vi "ATSh_SetTriggerDelay.vi"(10 "Delay":u32, 11 "Handle":u32) -> (0 "Return Code":u32, 3 "Handle_Out":u32)   [LabVIEW 2010]
doc: "_____AlazarTech, Scope_____\n\nConfigure the Trigger delay circuitry.\nHandle input."
uses:
  ATSApi.dll
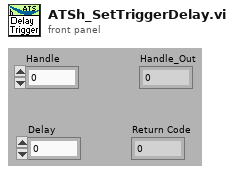
[diagram p1: front panel]
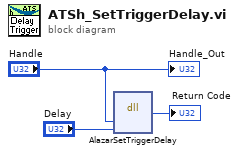
[diagram p0: block diagram]
diagram:
  n1 = dll-call lib="ATSApi.dll" fn="AlazarSetTriggerDelay"("h"="Handle", "Delay"="Delay") -> (→"Return Code":u32)  [unwired: 5 in, 2 out]
  "Handle_Out" <- "Handle"
